vi "Main software paths.vi"() -> (0 "templates dir path":path, 1 "data processing dir path":path, 2 "lv proc file path":path, 3 "LV project/exe dir path":path)   [LabVIEW 2020]
uses:
  external libraries/varilib/varilib.lvlib
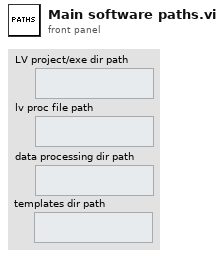
[diagram p1: front panel]
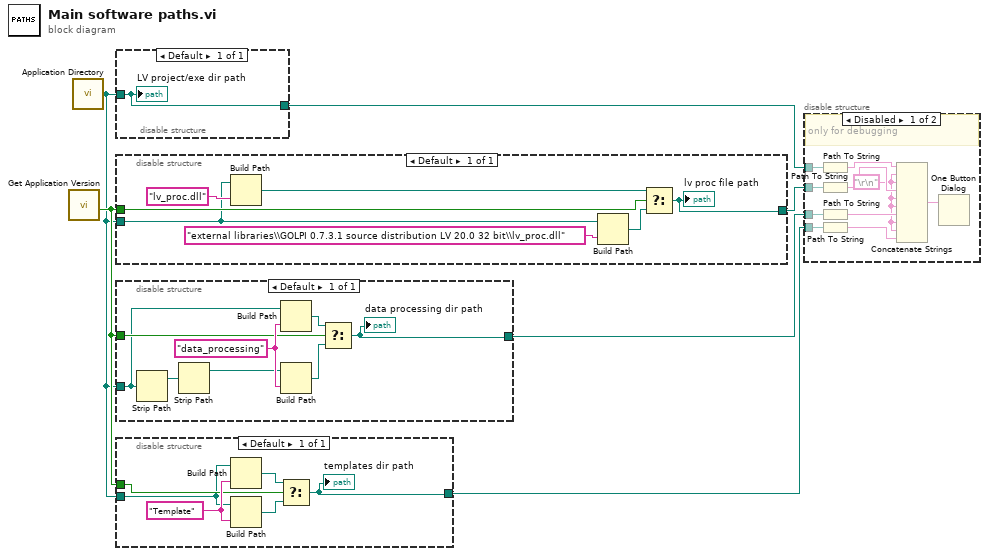
[diagram p0: block diagram]
diagram:
  n1 = call "Get Application Version.vi"() -> ("run time system"=w6:bool)  [unwired: 8 in, 3 out]
  n2 = call <vilib>:"Application Directory.vi"() -> ("Application Directory"=w1:path)
  n3 = disable-structure shown="Default" {
    disable-tunnel: [w7] -> w5
    disable-tunnel: w1 -> [w7]
    frame Enabled {
      "LV project/exe dir path" <- w7
    }
  }
  n4 = disable-structure shown="Default" {
    disable-tunnel: w6 -> [w10]
    disable-tunnel: [w9] -> w4
    disable-tunnel: w1 -> [w8]
    frame Enabled {
      n5 = Build Path(base path=w8, name or relative path="lv_proc.dll") -> (appended path=w11:path)
      n6 = Build Path(base path=w8, name or relative path="external libraries\\GOLPI 0.7.3.1 source distribution LV 20.0 32 bit\\lv_proc.dll") -> (appended path=w13:path)
      n7 = Select(t=w11, s=w10, f=w13) -> (s? t:f=w9:path)
      "lv proc file path" <- w9
    }
  }
  n8 = disable-structure shown="Default" {
    disable-tunnel: w6 -> [w19]
    disable-tunnel: [w18] -> w3
    disable-tunnel: w1 -> [w15]
    frame Enabled {
      w22 = "data_processing"
      n9 = Strip Path(path=w15) -> (stripped path=w17:path)  [unwired: 1 out]
      n10 = Strip Path(path=w17) -> (stripped path=w16:path)  [unwired: 1 out]
      n11 = Build Path(base path=w15, name or relative path=w22) -> (appended path=w21:path)
      n12 = Build Path(base path=w16, name or relative path=w22) -> (appended path=w20:path)
      n13 = Select(t=w21, s=w19, f=w20) -> (s? t:f=w18:path)
      "data processing dir path" <- w18
    }
  }
  n14 = disable-structure shown="Default" {
    disable-tunnel: w6 -> [w25]
    disable-tunnel: [w24] -> w2
    disable-tunnel: w1 -> [w23]
    frame Enabled {
      w28 = "Template"
      n15 = Build Path(base path=w23, name or relative path=w28) -> (appended path=w27:path)
      n16 = Build Path(base path=w23, name or relative path=w28) -> (appended path=w26:path)
      n17 = Select(t=w27, s=w25, f=w26) -> (s? t:f=w24:path)
      "templates dir path" <- w24
    }
  }
  n18 = disable-structure shown="Disabled" {
    disable-tunnel: w5 -> [w38 _]
    disable-tunnel: w4 -> [w36 _]
    disable-tunnel: w3 -> [w34 _]
    disable-tunnel: w2 -> [w32 _]
    frame Disabled {
      w29 = "\r\n"
      # "only for debugging"
      n19 = Path To String(path=w38) -> (string=w37:string)
      n20 = Path To String(path=w36) -> (string=w35:string)
      n21 = Path To String(path=w34) -> (string=w33:string)
      n22 = Path To String(path=w32) -> (string=w31:string)
      n23 = Concatenate Strings(w37, w29, w29, w35, w29, w29, w33, w29, w29, w31) -> (w30:string)
      n24 = One Button Dialog(message=w30) -> ()  [unwired: 1 in, 1 out]
    }
    frame Enabled {
    }
  }
